vi "Receive Write Bits Response.vi"(8 "error in (no error)":errorcluster, 11 "Port Selection Info":T1={"Port Name"="", "Amplifier Num"=1, "Baud Rate"=38400, "Char Formation"=enum."0"} {"Baud Rate" items=["38400"=38400, "19200"=19200, "9600"=9600, "115200"=0]; "Amplifier Num" max=31}) -> (0 "error out":errorcluster, 1 "Bits Num":u16=65535 format="%.0x", 2 "Address":u16=4102 format="%.0x", 3 "Port Selection Info Out":T1={"Port Name"="", "Amplifier Num"=1, "Baud Rate"=38400, "Char Formation"=enum."0"} {"Baud Rate" items=["38400"=38400, "19200"=19200, "9600"=9600, "115200"=0]; "Amplifier Num" max=31}, 4 "CRC Match":bool, 5 "FC":u8=3, 7 "Bank":u8)   [LabVIEW 2014, in "ALPHA5 RS485.lvlib"]
uses:
  ALPHA5 RS485.lvlib
  typedefs/Port Selection Info.ctl
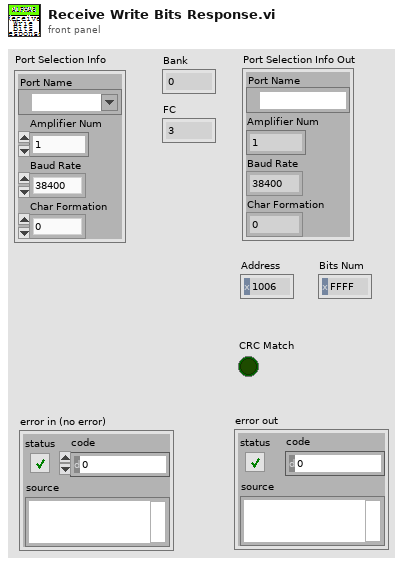
[diagram p1: front panel]
types:
  T1 = typedef "ALPHA5 RS485.lvlib/Port Selection Info.ctl" = cluster{"Port Name":refnum<visa-resource-name>, "Amplifier Num":u8, "Baud Rate":u32, "Char Formation":enum16{"0", "1", "2", "3", "4", "5"}}
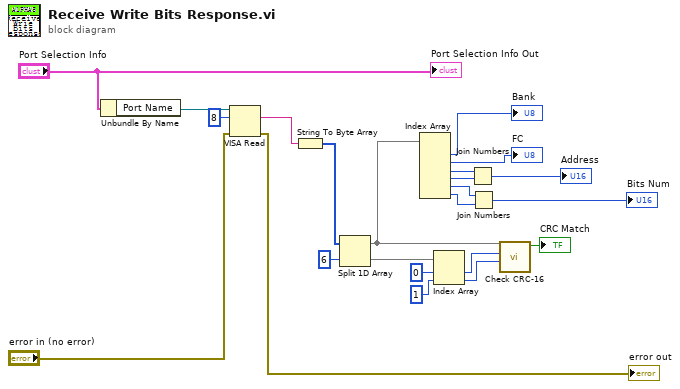
[diagram p0: block diagram]
diagram:
  n1 = Unbundle By Name("Port Selection Info") -> ("Port Name"=w22:refnum<visa-resource-name>)
  n2 = VISA Read(VISA resource name=w22, byte count=u32 8, error in (no error)="error in (no error)") -> (read buffer=w19:string, error out=→"error out":errorcluster)  [unwired: 2 out]
  n3 = String To Byte Array(string=w19) -> (unsigned byte array=w10:u8[])
  n4 = Split 1D Array(array=w10, index=6) -> (first subarray=w3:u8[], second subarray=w5:u8[])
  n5 = Index Array(array=w3) -> (element #1=→"Bank":u8, element #2=→"FC":u8, element #3=w16:u8, element #4=w15:u8, element #5=w13:u8, element #6=w12:u8)  [unwired: 6 in]
  n6 = Index Array(array=w5, index #1=0 ("index"), index #2=1 ("index")) -> (element #1=w4:u8, element #2=w6:u8)
  n7 = Join Numbers(hi=w16, lo=w15) -> ((hi.lo)=→"Address":u16)
  n8 = Join Numbers(hi=w13, lo=w12) -> ((hi.lo)=→"Bits Num":u16)
  n9 = call "Check CRC-16.vi"("CRC-16-H"=w6, "CRC-16-L"=w4, "Data In"=w3) -> ("Check Result"=→"CRC Match":bool)  [unwired: 7 in, 1 out]
  "Port Selection Info Out" <- "Port Selection Info"
